vi "calculate_T1_curve.vi"(8 "normalise":enum16{"No normalise", "Minimum", "Same pulse"}(ring), 9 "T1_parameters":T1, 10 "triggers":u32[][](array[numeric]), 11 "timetags":u32[][](array[numeric])) -> (3 "T1_curve_out":cluster{"dark_time_us":dbl[], "PL_signal":dbl[]})   [LabVIEW 2014]
panel:
  in  "norm_start_us":dbl
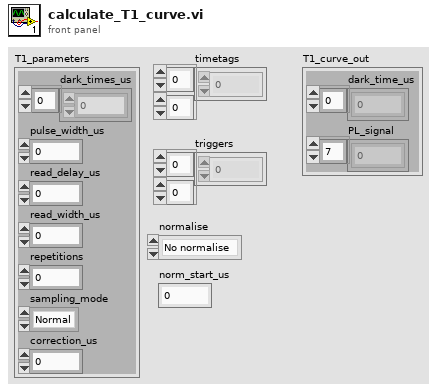
[diagram p1: front panel]
types:
  T1 = cluster{"dark_times_us":dbl[], "pulse_width_us":dbl, "read_delay_us":dbl, "read_width_us":dbl, "repetitions":i32, "sampling_mode":enum16{"Normal", "Sweep"}, "correction_us":dbl}
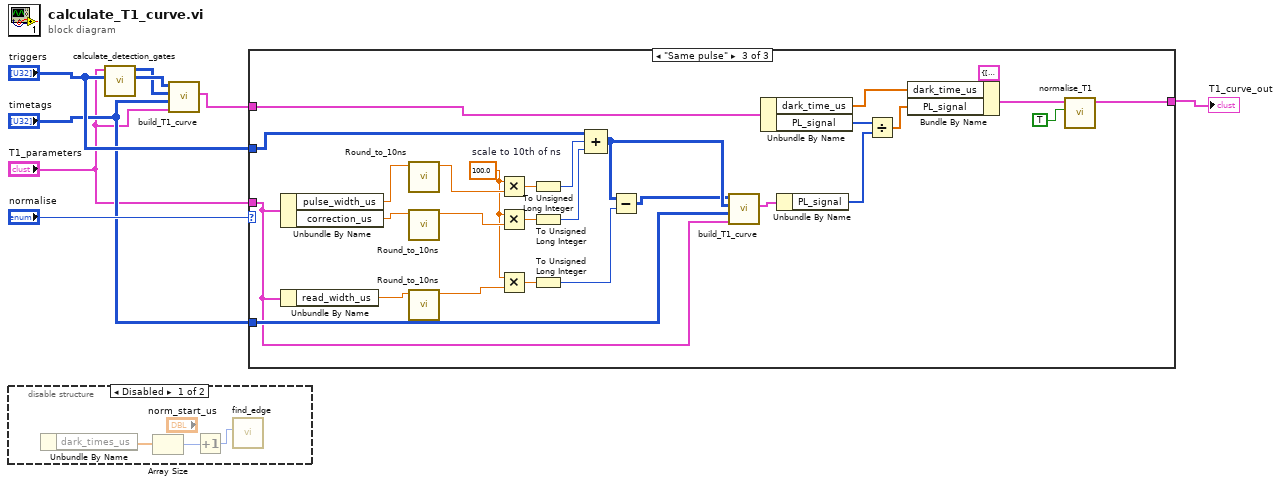
[diagram p0: block diagram]
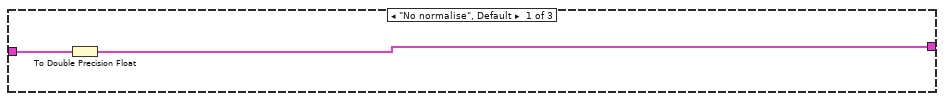
[diagram p3: hidden frame]
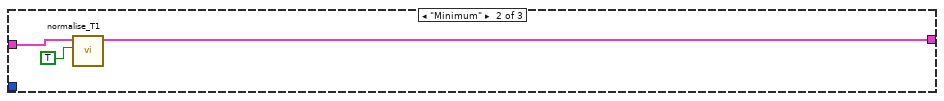
[diagram p4: hidden frame]
diagram:
  n1 = disable-structure shown="Disabled" {
    frame Disabled {
      n2 = Unbundle By Name() -> ("dark_times_us"=w10:dbl[])  [unwired: 1 in]
      n3 = Array Size(array=w10) -> (size(s)=w9:i32)
      n4 = Increment(x=w9) -> (x+1=w11:i32)
      n5 = call "find_edge.vi"("q_pulses"=w11) -> ()  [unwired: 11 in]
    }
    frame Enabled {
    }
  }
  n6 = call "calculate_detection_gates.vi"("triggers"="triggers", "T1_parameters"="T1_parameters") -> ("start_read"=w4:u32[][], "stop_read"=w3:u32[][])  [unwired: 8 in]
  n7 = call "build_T1_curve.vi"("T1_parameters"="T1_parameters", "timetags"="timetags", "stop_read"=w3, "start_read"=w4) -> ("T1 curve"=w5:cluster{"dark_time_us":dbl[], "PL_signal":i32[]})  [unwired: 5 in, 2 out]
  n8 = case shown="\"Same pulse\"" "normalise" {
    tunnel: [w12 w16 w29] -> w7
    tunnel: w5 -> [w13 w15 w35]
    tunnel: "T1_parameters" -> [_ _ w25]
    tunnel: "triggers" -> [_ _ w40]
    tunnel: "timetags" -> [_ _ w26]
    frame "No normalise", Default {
      n9 = To Double Precision Float(number=w13) -> (double precision float=w12:cluster{"dark_time_us":dbl[], "PL_signal":dbl[]})
    }
    frame "Minimum" {
      n10 = call "normalise_T1.vi"("normalise"=TRUE, "T1_curve_in"=w15) -> ("T1_curve_out"=w16:cluster{"dark_time_us":dbl[], "PL_signal":dbl[]})  [unwired: 9 in]
    }
    frame "Same pulse" {
      w17 = 100.0  # scale to 10th of ns
      n11 = Unbundle By Name(w25) -> ("pulse_width_us"=w42:dbl, "correction_us"=w21:dbl)
      n12 = Unbundle By Name(w25) -> ("read_width_us"=w23:dbl)
      n13 = call "Round_to_10ns.vi"("time_us"=w42) -> ("rounded_us"=w43:dbl)  [unwired: 10 in]
      n14 = call "Round_to_10ns.vi"("time_us"=w21) -> ("rounded_us"=w19:dbl)  [unwired: 10 in]
      n15 = call "Round_to_10ns.vi"("time_us"=w23) -> ("rounded_us"=w22:dbl)  [unwired: 10 in]
      n16 = Multiply(x=w17, y=w43) -> (x*y=w44:dbl)
      n17 = Multiply(x=w17, y=w19) -> (x*y=w20:dbl)
      n18 = Multiply(x=w17, y=w22) -> (x*y=w39:dbl)
      n19 = To Unsigned Long Integer(number=w44) -> (unsigned 32bit integer=w41:u32)
      n20 = To Unsigned Long Integer(number=w20) -> (unsigned 32bit integer=w18:u32)
      n21 = To Unsigned Long Integer(number=w39) -> (unsigned 32bit integer=w38:u32)
      n22 = Compound Arithmetic op=ADD(w40, w41, w18) -> (w28:u32[][])
      n23 = Subtract(x=w28, y=w38) -> (x-y=w27:u32[][])
      n24 = call "build_T1_curve.vi"("T1_parameters"=w25, "timetags"=w26, "stop_read"=w28, "start_read"=w27) -> ("T1 curve"=w24:cluster{"dark_time_us":dbl[], "PL_signal":i32[]})  [unwired: 5 in, 2 out]
      n25 = Unbundle By Name(w35) -> ("dark_time_us"=w32:dbl[], "PL_signal"=w37:i32[])
      n26 = Unbundle By Name(w24) -> ("PL_signal"=w36:i32[])
      n27 = Divide(x=w37, y=w36) -> (x/y=w33:dbl[])
      n28 = Bundle By Name(cluster=cluster{"dark_time_us":dbl[], "PL_signal":dbl[]} {"dark_time_us"=[0.0, 0.224, 0.25, 0.278, 0.31, 0.346, 0.386, 0.43, 0.48, 0.536, 0.598, 0.666, 0.742, 0.828, 0.924, 1.03, 1.15, 1.282, 1.43, 1.596, 1.78, 1.986, 2.214, 2.47, 2.756, 3.074, 3.428, 3.824, 4.266, 4.76, 5.308, 5.922, 6.606, 7.368, 8.22, 9.168, 10.228, 11.408, 12.726, 14.196, 15.834, 17.664, 19.704, 21.978, 24.518, 27.348, 30.506, 34.03, 37.96, 42.344, 47.234, 52.688, 58.774, 65.56, 73.132, 81.578, 90.998, 101.508, 113.23, 126.308, 140.894, 157.166, 175.316, 195.562, 218.146, 243.34, 271.442, 302.79, 337.758, 376.764, 420.276, 468.812, 522.954, 583.348, 650.716, 725.866, 809.692, 903.202, 1007.51, 1123.862, 1253.654, 1398.434, 1559.934, 1740.086, 1941.042, 2165.206, 2415.258, 2694.188, 3005.33, 3352.406, 3739.564, 4171.434, 4653.178, 5190.558, 5789.996, 6458.664, 7204.552, 8036.582, 8964.698, 10000.0], "PL_signal"=[0.0, 30162.0, 30216.0, 30271.0, 30447.0, 30194.0, 29950.0, 30205.0, 29749.0, 30023.0, 29910.0, 30178.0, 29557.0, 29963.0, 29874.0, 29745.0, 29693.0, 29416.0, 29426.0, 28896.0, 29404.0, 29579.0, 29329.0, 29301.0, 29319.0, 29336.0, 29020.0, 28949.0, 28673.0, 28851.0, 28786.0, 28905.0, 28773.0, 28800.0, 28895.0, 28979.0, 28792.0, 28721.0, 28833.0, 29038.0, 28609.0, 28428.0, 28816.0, 28747.0, 28606.0, 28634.0, 28218.0, 28663.0, 28387.0, 28417.0, 28387.0, 28245.0, 28148.0, 28314.0, 28438.0, 28288.0, 28273.0, 28233.0, 27988.0, 28029.0, 27940.0, 27978.0, 27871.0, 27726.0, 27604.0, 27716.0, 27751.0, 27819.0, 27634.0, 27627.0, 27429.0, 27224.0, 27355.0, 27321.0, 27045.0, 27385.0, 27119.0, 27202.0, 26619.0, 26846.0, 26937.0, 26934.0, 26829.0, 27113.0, 27054.0, 26996.0, 26631.0, 26915.0, 26931.0, 26875.0, 26787.0, 26555.0, 26904.0, 26696.0, 26648.0, 26782.0, 26783.0, 26948.0, 26935.0, 26747.0]} ("T1_curve_out"), "dark_time_us"=w32, "PL_signal"=w33) -> (w30:cluster{"dark_time_us":dbl[], "PL_signal":dbl[]})
      n29 = call "normalise_T1.vi"("normalise"=TRUE, "T1_curve_in"=w30) -> ("T1_curve_out"=w29:cluster{"dark_time_us":dbl[], "PL_signal":dbl[]})  [unwired: 9 in]
    }
  }
  "T1_curve_out" <- w7
